vi "Modify G08.vi"(7 "DG Number":i32, 8 "error in (no error)":errorcluster, 11 "Settings 2":T1={"Channel A"={"Delay (µs)"=0.013000000000000001, "Pulse Width (µs)"=0.019, "Output Modulo"=300, "Output Offset"=0, "Go Signal"=16, "Polarity"=TRUE, "Terminate"=FALSE}, "Channel B"={"Delay (µs)"=0.032, "Pulse Width (µs)"=0.019, "Output Modulo"=300, "Output Offset"=0, "Go Signal"=16, "Polarity"=TRUE, "Terminate"=FALSE}, "Channel C"={"Delay (µs)"=0.0, "Pulse Width (µs)"=0.01, "Output Modulo"=300, "Output Offset"=0, "Go Signal"=16, "Polarity"=TRUE, "Terminate"=FALSE}, "Channel D"={"Delay (µs)"=0.01, "Pulse Width (µs)"=0.01, "Output Modulo"=300, "Output Offset"=0, "Go Signal"=16, "Polarity"=TRUE, "Terminate"=FALSE}, "Channel E"={"Delay (µs)"=0.039999999999999994, "Pulse Width (µs)"=0.01, "Output Modulo"=300, "Output Offset"=1, "Go Signal"=16, "Polarity"=TRUE, "Terminate"=FALSE, "Disconnect"=FALSE, "Onto MsBus"=FALSE, "Input Positive"=TRUE}, "Channel F"={"Delay (µs)"=0.04999999999999999, "Pulse Width (µs)"=0.01, "Output Modulo"=300, "Output Offset"=1, "Go Signal"=16, "Polarity"=TRUE, "Terminate"=FALSE, "Disconnect"=FALSE, "Onto MsBus"=FALSE, "Input Positive"=TRUE}, "Clock Enable"=TRUE, "Ocillator Divider"=2, "Trigger Divider"=1, "Trigger Multiplier"=4, "Clock Source"=3, "Trigger Terminate"=TRUE, "Gate Terminate"=TRUE, "Trigger Level"=0.2, "Gate Level"=0.0, "Gate Delay (µs)"=-1.0, "MS Bus"=1, "Internal Clock (µs)"=0.0083333, "Stop Trigger"=1, "Gate Divider"=0, "Force Trigger (µs)"=-1.0, "Step Back Time (µs)"=-1.0, "Burst Counter"=1, "Positive Gate"=TRUE, "Trigger Source"=TRUE, "Gate Type"=TRUE, "Synchronize Gate"=FALSE, "Trigger Slope"=TRUE, "Stop on Preset"=FALSE, "Reset When Done"=TRUE, "Trigger Enable"=TRUE, "Gate AB"=0, "Gate CD"=0, "Gate EF"=0} {"Gate EF" items=["Normal"=0, "EF_OR"=1048576, "EF_AND"=2097152, "EF_XOR"=3145728]; "Gate CD" items=["Normal"=0, "CD_OR"=262144, "CD_AND"=524288, "CD_XOR"=786432]; "Gate AB" items=["Normal"=0, "AB_OR"=65536, "AB_AND"=131072, "AB_XOR"=196608]; "Step Back Time (µs)" min=-1.0 format="%.6f"; "Force Trigger (µs)" min=-1.0 format="%.6f"; "Gate Delay (µs)" min=-1.0 format="%.6f"; "Internal Clock (µs)" min=0.0 format="%.6f"; "MS Bus" format="%04x" items=["Local Primary"=1, "Local Secondary"=2, "Local Force"=4, "Resynchronize"=8, "Master Primary"=16, "Master Secondary"=32, "Master Force"=64, "System Clock"=128, "Delay Clock"=256, "Inhibit Local"=512, "Start Local"=1024, "Start Bus"=2048, "Step Back Local"=4096, "Step Back Bus"=8192, "Enable From E"=65536, "Enable From F"=131072, "Enable From Bus"=262144]; "Gate Level" min=-2.5 max=2.5 format="%.3g"; "Trigger Level" min=-2.5 max=2.5 format="%.3f"; "Clock Source" items=["Internal Oscillator"=1, "External Trigger"=2, "Trigger & Oscillator"=3, "Master Slave Bus"=4]; "Trigger Multiplier" min=1; "Trigger Divider" min=1; "Ocillator Divider" min=1; "Channel F"."Go Signal" format="%04x" items=["Loc Prim"=1, "Loc Sec"=2, "Loc Force"=4, "Resynch"=8, "Mas Prim"=16, "Mas Sec"=32, "Mas Force"=64, "Sys Clock"=128, "Delay Clock"=256, "Inhibit Local"=512, "Start Local"=1024, "Start Bus"=2048, "Step Back Loc"=4096, "Step Back Bus"=8192, "From E"=65536, "From F"=131072, "From Bus"=262144]; "Channel F"."Pulse Width (µs)" min=0.0 max=8947840.0 format="%.6f"; "Channel F"."Delay (µs)" min=0.0 format="%.6f"; "Channel E"."Go Signal" format="%04x" items=["Loc Prim"=1, "Loc Sec"=2, "Loc Force"=4, "Resynch"=8, "Mas Prim"=16, "Mas Sec"=32, "Mas Force"=64, "Sys Clock"=128, "Delay Clock"=256, "Inhibit Local"=512, "Start Local"=1024, "Start Bus"=2048, "Step Back Loc"=4096, "Step Back Bus"=8192, "From E"=65536, "From F"=131072, "From Bus"=262144]; "Channel E"."Pulse Width (µs)" min=0.0 max=8947840.0 format="%.6f"; "Channel E"."Delay (µs)" min=0.0 format="%.6f"; "Channel D"."Go Signal" format="%04x" items=["Loc Prim"=1, "Loc Sec"=2, "Loc Force"=4, "Resynch"=8, "Mas Prim"=16, "Mas Sec"=32, "Mas Force"=64, "Sys Clock"=128, "Delay Clock"=256, "Inhibit Local"=512, "Start Local"=1024, "Start Bus"=2048, "Step Back Loc"=4096, "Step Back Bus"=8192, "From E"=65536, "From F"=131072, "From Bus"=262144]; "Channel D"."Pulse Width (µs)" min=0.0 max=8947840.0 format="%.6f"; "Channel D"."Delay (µs)" min=0.0 format="%.6f"; "Channel C"."Go Signal" format="%04x" items=["Loc Prim"=1, "Loc Sec"=2, "Loc Force"=4, "Resynch"=8, "Mas Prim"=16, "Mas Sec"=32, "Mas Force"=64, "Sys Clock"=128, "Delay Clock"=256, "Inhibit Local"=512, "Start Local"=1024, "Start Bus"=2048, "Step Back Loc"=4096, "Step Back Bus"=8192, "From E"=65536, "From F"=131072, "From Bus"=262144]; "Channel C"."Pulse Width (µs)" min=0.0 max=8947840.0 format="%.6f"; "Channel C"."Delay (µs)" min=0.0 format="%.6f"; "Channel B"."Go Signal" format="%04x" items=["Loc Prim"=1, "Loc Sec"=2, "Loc Force"=4, "Resynch"=8, "Mas Prim"=16, "Mas Sec"=32, "Mas Force"=64, "Sys Clock"=128, "Delay Clock"=256, "Inhibit Local"=512, "Start Local"=1024, "Start Bus"=2048, "Step Back Loc"=4096, "Step Back Bus"=8192, "From E"=65536, "From F"=131072, "From Bus"=262144]; "Channel B"."Pulse Width (µs)" min=0.0 max=8947840.0 format="%.6f"; "Channel B"."Delay (µs)" min=0.0 format="%.6f"; "Channel A"."Go Signal" format="%04x" items=["Loc Prim"=1, "Loc Sec"=2, "Loc Force"=4, "Resynch"=8, "Mas Prim"=16, "Mas Sec"=32, "Mas Force"=64, "Sys Clock"=128, "Delay Clock"=256, "Inhibit Local"=512, "Start Local"=1024, "Start Bus"=2048, "Step Back Loc"=4096, "Step Back Bus"=8192, "From E"=65536, "From F"=131072, "From Bus"=262144]; "Channel A"."Pulse Width (µs)" min=0.0 max=8947840.0 format="%.6f"; "Channel A"."Delay (µs)" min=0.0 format="%.6f"}) -> (0 "error out":errorcluster)   [LabVIEW 2009, in "POLARIS BME DG.lvlib"]
doc: "long Set_BME_G05(double FireFirst_T0, unsigned long OutputModulo_T0, BOOL Active_T0, BOOL Positive_T0, BOOL Terminate_T0, BOOL HighDrive_T0, double FireFirst_A, unsigned long OutputModulo_A, BOOL Active_A, BOOL Positive_A, BOOL Terminate_A, BOOL HighDrive_A, double FireFirst_B, unsigned long OutputModulo_B, BOOL Active_B, BOOL Positive_B, BOOL Terminate_B, BOOL HighDrive_B, BOOL Gate_AB, unsigned long OutputLevel, BOOL TriggerTerminate, BOOL ClockEnable, double InternalClock, double TriggerLevel, unsigned long PresetValue, unsigned long DivideBy, unsigned long ClockSource, unsigned long GateDivider, BOOL PositiveGate, BOOL InternalTrigger, BOOL InternalArm, BOOL SoftwareTrigger, BOOL RisingEdge, BOOL StopOnPreset, BOOL ResetWhenDone, BOOL TriggerEnable, long DG_Number);"
uses:
  POLARIS BME DG.lvlib
  Settings G08.ctl
  BME DLL/DelayGenerator.dll
panel:
  # "NOTICE -- YOU MUST LEAVE THIS NOTICE IN PLACE.  PER THE TERMS OF THE LICENSE BELOW, YOU MAY SUBLICENSE THIS SOFTWARE \nIN ANY WAY THAT DOES NOT CONFLICT WITH THIS LICENSE.\n\n### BSD License (http://www.opensource.org/licenses/bsd-license.php) Begin ###\n \nCopyright (c) 2011, Applied Energetics, http://www.appliedenergetics.com,\n                               Richard Schwerdtfeger, <rschwerdtfeger@appliedenergetics.com>\n\nAll rights reserved.\n\nRedistribution and use in source and binary forms, with or without modification, are permitted provided that the \nfollowing conditions are met:\n\n    * Redistributions of source code must retain the above copyright notice, this list of conditions and the following disclaimer.\n    * Redistributions in binary form must reproduce the above copyright notice, this list of conditions and the following disclaimer \n       in the documentation and/or other materials provided with the distribution.\n    * Neither the name of Richard Schwerdtfeger, Applied Energetics, Inc., nor the names of its contributors may be used to \n       endorse or promote products derived from this software without specific prior written permission.\n\nTHIS SOFTWARE IS PROVIDED BY THE COPYRIGHT HOLDERS AND CONTRIBUTORS \"AS IS\" AND ANY EXPRESS OR IMPLIED WARRANTIES, \nINCLUDING, BUT NOT LIMITED TO, THE IMPLIED WARRANTIES OF MERCHANTABILITY AND FITNESS FOR A PARTICULAR PURPOSE ARE \nDISCLAIMED. IN NO EVENT SHALL THE COPYRIGHT OWNER OR CONTRIBUTORS BE LIABLE FOR ANY DIRECT, INDIRECT, INCIDENTAL,\n SPECIAL, EXEMPLARY, OR CONSEQUENTIAL DAMAGES (INCLUDING, BUT NOT LIMITED TO, PROCUREMENT OF SUBSTITUTE GOODS OR \nSERVICES; LOSS OF USE, DATA, OR PROFITS; OR BUSINESS INTERRUPTION) HOWEVER CAUSED AND ON ANY THEORY OF LIABILITY, \nWHETHER IN CONTRACT, STRICT LIABILITY, OR TORT (INCLUDING NEGLIGENCE OR OTHERWISE) ARISING IN ANY WAY OUT OF THE USE \nOF THIS SOFTWARE, EVEN IF ADVISED OF THE POSSIBILITY OF SUCH DAMAGE.\n\n### BSD License End ###"
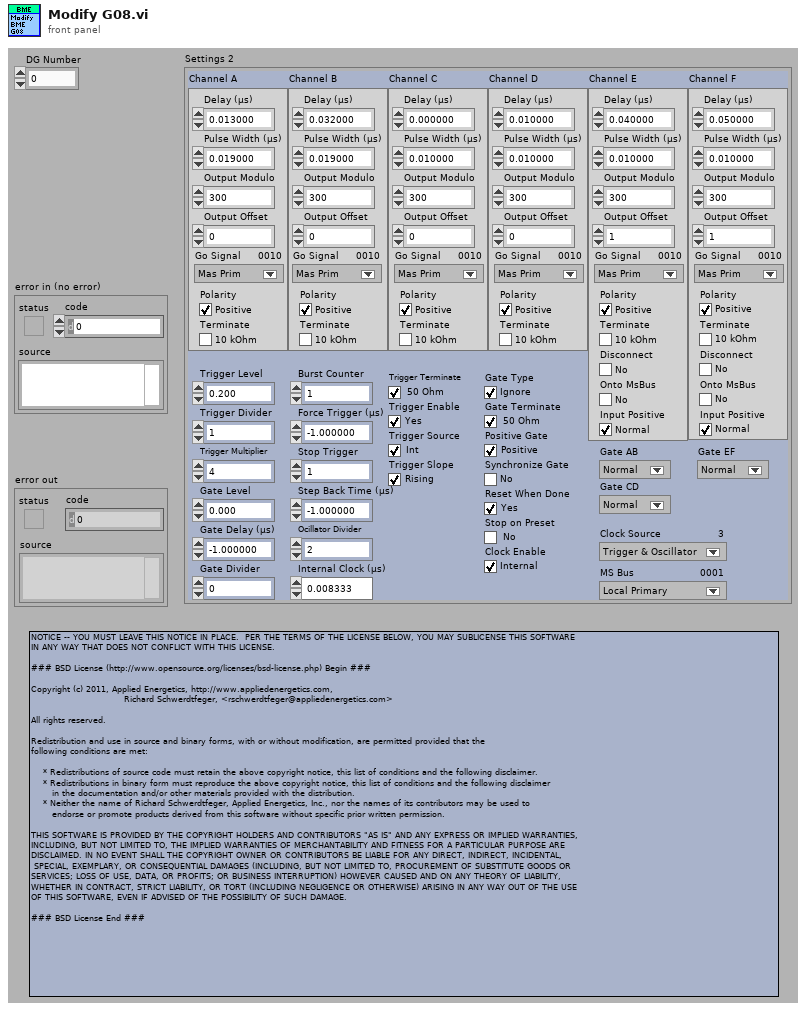
[diagram p1: front panel]
types:
  T1 = typedef "POLARIS BME DG.lvlib/Settings G08.ctl" = cluster{"Channel A":cluster{"Delay (µs)":dbl, "Pulse Width (µs)":dbl, "Output Modulo":u32, "Output Offset":u32, "Go Signal":u32, "Polarity":bool, "Terminate":bool}, "Channel B":cluster{"Delay (µs)":dbl, "Pulse Width (µs)":dbl, "Output Modulo":u32, "Output Offset":u32, "Go Signal":u32, "Polarity":bool, "Terminate":bool}, "Channel C":cluster{"Delay (µs)":dbl, "Pulse Width (µs)":dbl, "Output Modulo":u32, "Output Offset":u32, "Go Signal":u32, "Polarity":bool, "Terminate":bool}, "Channel D":cluster{"Delay (µs)":dbl, "Pulse Width (µs)":dbl, "Output Modulo":u32, "Output Offset":u32, "Go Signal":u32, "Polarity":bool, "Terminate":bool}, "Channel E":cluster{"Delay (µs)":dbl, "Pulse Width (µs)":dbl, "Output Modulo":u32, "Output Offset":u32, "Go Signal":u32, "Polarity":bool, "Terminate":bool, "Disconnect":bool, "Onto MsBus":bool, "Input Positive":bool}, "Channel F":cluster{"Delay (µs)":dbl, "Pulse Width (µs)":dbl, "Output Modulo":u32, "Output Offset":u32, "Go Signal":u32, "Polarity":bool, "Terminate":bool, "Disconnect":bool, "Onto MsBus":bool, "Input Positive":bool}, "Clock Enable":bool, "Ocillator Divider":u32, "Trigger Divider":u32, "Trigger Multiplier":u32, "Clock Source":u32, "Trigger Terminate":bool, "Gate Terminate":bool, "Trigger Level":dbl, "Gate Level":dbl, "Gate Delay (µs)":dbl, "MS Bus":u32, "Internal Clock (µs)":dbl, "Stop Trigger":u32, "Gate Divider":u32, "Force Trigger (µs)":dbl, "Step Back Time (µs)":dbl, "Burst Counter":u32, "Positive Gate":bool, "Trigger Source":bool, "Gate Type":bool, "Synchronize Gate":bool, "Trigger Slope":bool, "Stop on Preset":bool, "Reset When Done":bool, "Trigger Enable":bool, "Gate AB":u32, "Gate CD":u32, "Gate EF":u32}
  T2 = cluster{"Delay (µs)":dbl, "Pulse Width (µs)":dbl, "Output Modulo":u32, "Output Offset":u32, "Go Signal":u32, "Polarity":bool, "Terminate":bool}
  T3 = cluster{"Delay (µs)":dbl, "Pulse Width (µs)":dbl, "Output Modulo":u32, "Output Offset":u32, "Go Signal":u32, "Polarity":bool, "Terminate":bool, "Disconnect":bool, "Onto MsBus":bool, "Input Positive":bool}
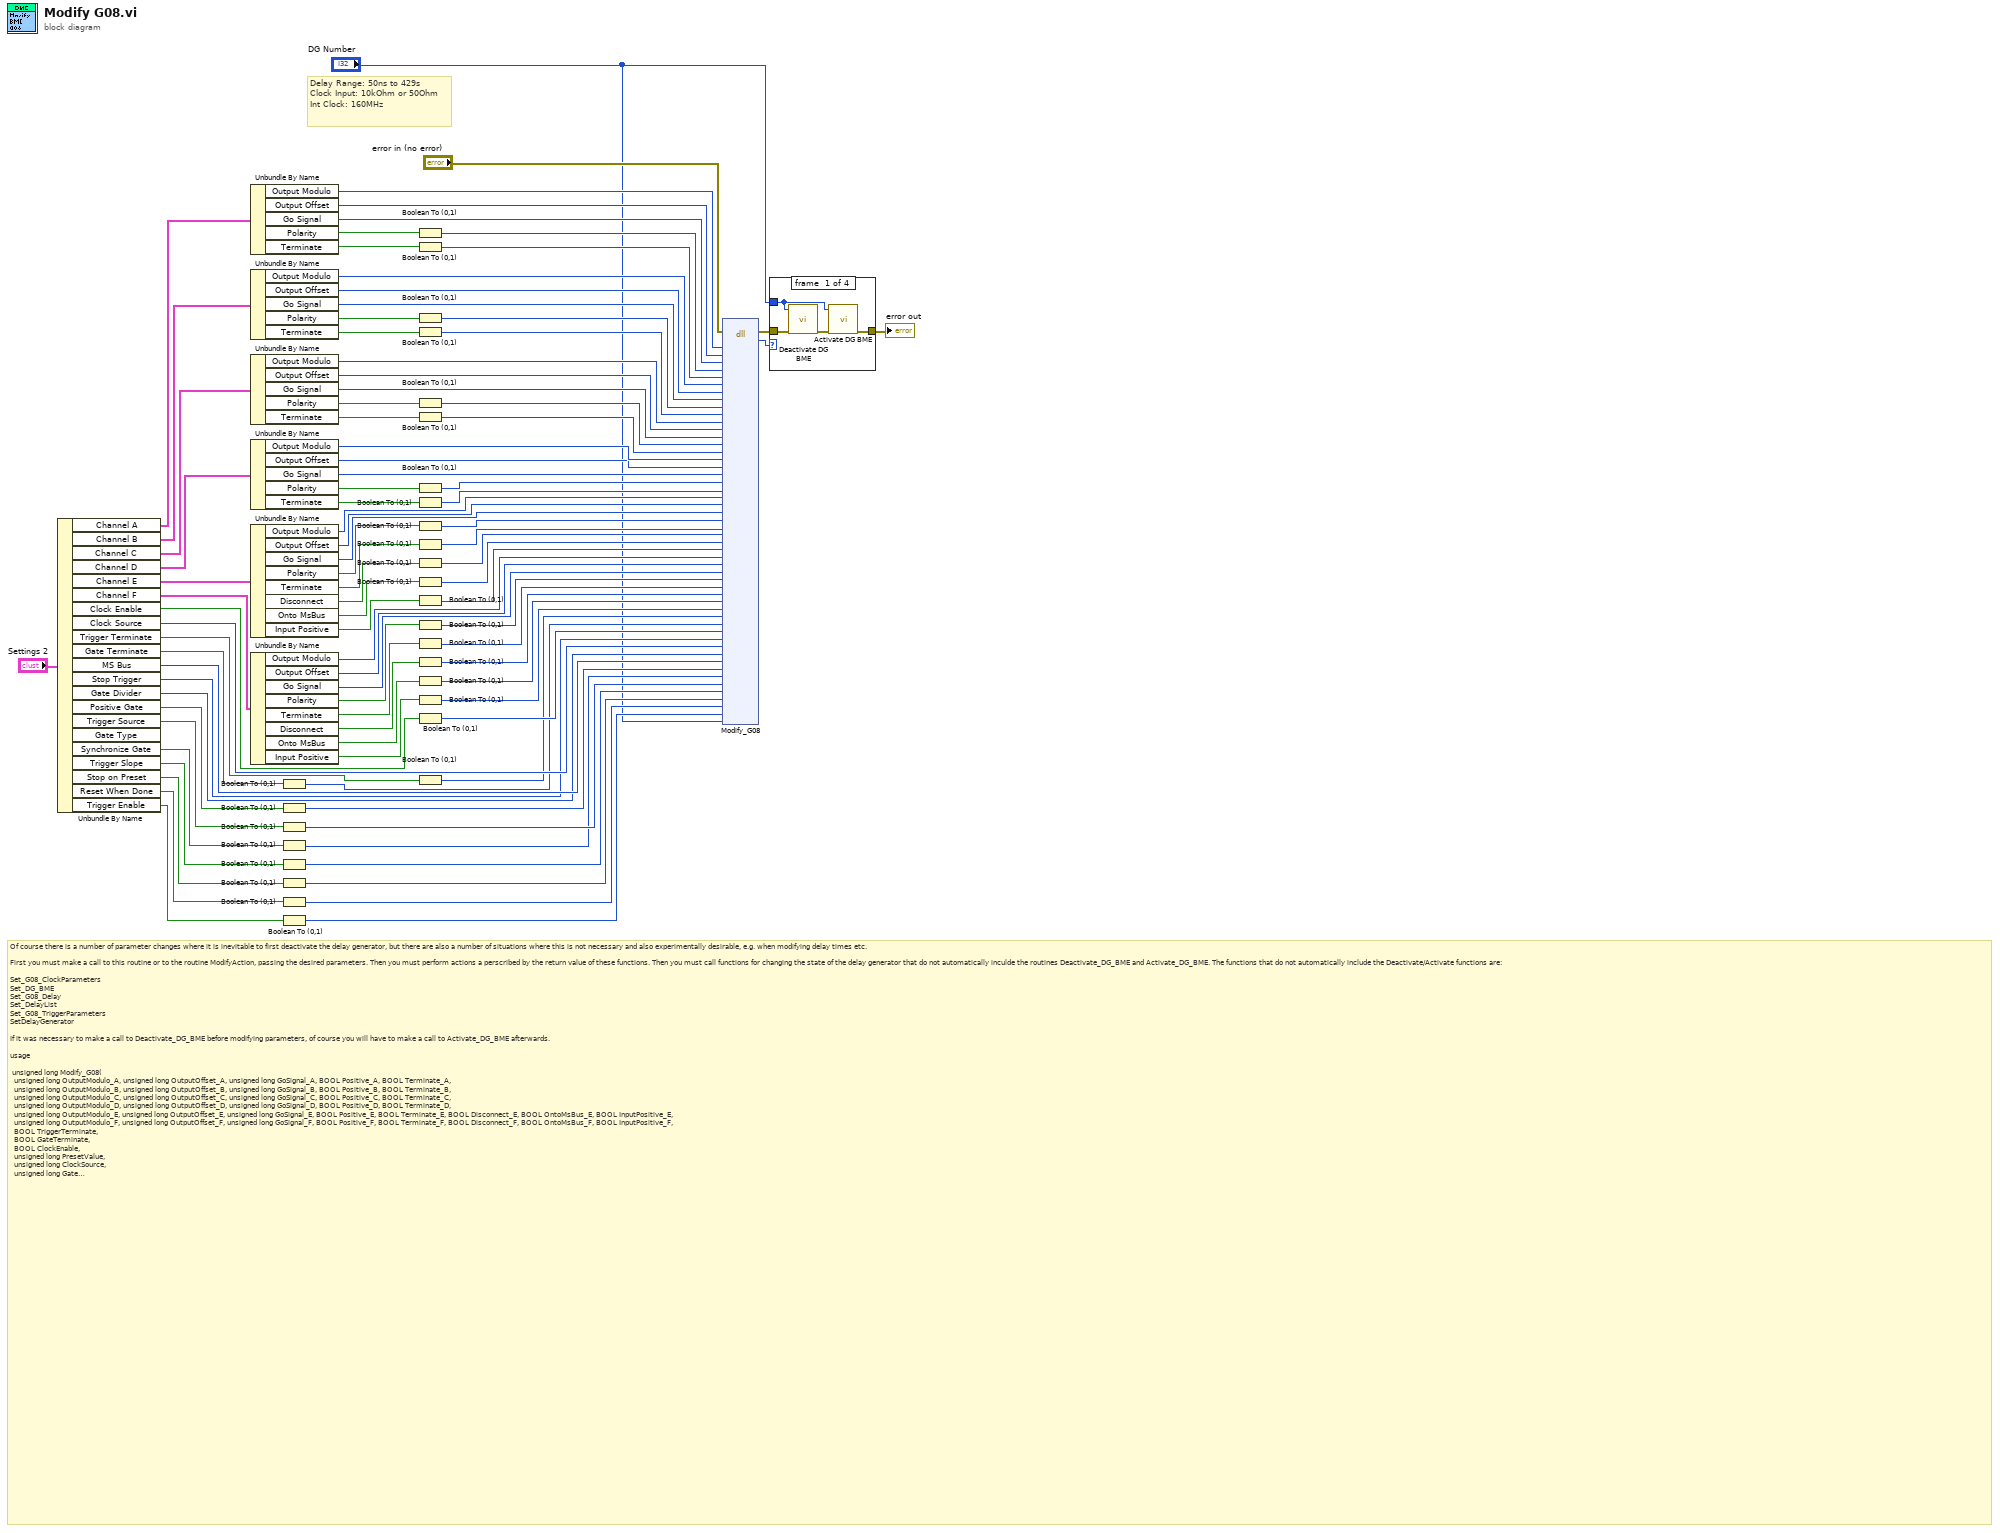
[diagram p0: block diagram]
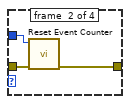
[diagram p2: hidden frame]
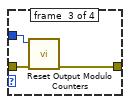
[diagram p3: hidden frame]
diagram:
  # "Delay Range: 50ns to 429s\nClock Input: 10kOhm or 50Ohm\nInt Clock: 160MHz"
  # "Of course there is a number of parameter changes where it is inevitable to first deactivate the delay generator, but there are also a number of situations where this is not necessary and also experimentally desirable, e.g. when modifying delay times etc. \n\nFirst you must make a call to this routine or to the routine ModifyAction, passing the desired parameters. Then you must perform actions a perscribed by the return value of these functions. Then you must call functions for changing the state of the delay generator that do not automatically inculde the routines Deactivate_DG_BME and Activate_DG_BME. The functions that do not automatically include the Deactivate/Activate functions are:\n\nSet_G08_ClockParameters\nSet_DG_BME\nSet_G08_Delay\nSet_DelayList\nSet_G08_TriggerParameters\nSetDelayGenerator\n\nIf it was necessary to make a call to Deactivate_DG_BME before modifying parameters, of course you will have to make a call to Activate_DG_BME afterwards.\n\nusage\n\n\tunsigned long Modify_G08(\n\t\tunsigned long OutputModulo_A, unsigned long OutputOffset_A, unsigned long GoSignal_A, BOOL Positive_A, BOOL Terminate_A,\n\t\tunsigned long OutputModulo_B, unsigned long OutputOffset_B, unsigned long GoSignal_B, BOOL Positive_B, BOOL Terminate_B,\n\t\tunsigned long OutputModulo_C, unsigned long OutputOffset_C, unsigned long GoSignal_C, BOOL Positive_C, BOOL Terminate_C,\n\t\tunsigned long OutputModulo_D, unsigned long OutputOffset_D, unsigned long GoSignal_D, BOOL Positive_D, BOOL Terminate_D,\n\t\tunsigned long OutputModulo_E, unsigned long OutputOffset_E, unsigned long GoSignal_E, BOOL Positive_E, BOOL Terminate_E, BOOL Disconnect_E, BOOL OntoMsBus_E, BOOL InputPositive_E, \n\t\tunsigned long OutputModulo_F, unsigned long OutputOffset_F, unsigned long GoSignal_F, BOOL Positive_F, BOOL Terminate_F, BOOL Disconnect_F, BOOL OntoMsBus_F, BOOL InputPositive_F, \n\t\tBOOL TriggerTerminate, \n\t\tBOOL GateTerminate, \n\t\tBOOL ClockEnable,\n\t\tunsigned long PresetValue,\n\t\tunsigned long ClockSource, \n\t\tunsigned long GateDivider,\n\t\tunsigned long MS_Bus, \n\t\tBOOL PositiveGate, \n\t\tBOOL SynchronizeGate,\n\t\tBOOL InternalTrigger, \n\t\tBOOL RisingEdge, \n\t\tBOOL StopOnPreset,\n\t\tBOOL ResetWhenDone, \n\t\tBOOL TriggerEnable, \n\t\tlong DG_Number);\n\nparameters\n\n\tSee the above named routines, e.g. Set_G08_TriggerParameters for a description of the parameters. Note that this routine does not pass the complete set of parameters, since for some parameters there is no action necessary under any situation.\n\nreturn value\n\n\tThe return value of this function indicates the actions that are also necessary when the specified parameters are to be set. Each bit in the return value specifies an action that should be performed:\n\tBit 0 True:  it is necessary to call the routine Deactivate_DG_BME before actually calling the routine SetDelayGenerator.\n\tBit 1 True:  it is necessary to call the routine ResetEventCounter.\n\tBit 2 True:  it is necessary to call the routine ResetOutputModuloCounters."
  n1 = Unbundle By Name("Settings 2") -> ("Channel A"=w80:T2, "Channel B"=w67:T2, "Channel C"=w66:T2, "Channel D"=w65:T2, "Channel E"=w64:T3, "Channel F"=w63:T3, "Clock Enable"=w81:bool, "Clock Source"=w31:u32, "Trigger Terminate"=w82:bool, "Gate Terminate"=w83:bool, "MS Bus"=w28:u32, "Stop Trigger"=w27:u32, "Gate Divider"=w26:u32, "Positive Gate"=w84:bool, "Trigger Source"=w85:bool, "Synchronize Gate"=w86:bool, "Trigger Slope"=w87:bool, "Stop on Preset"=w88:bool, "Reset When Done"=w89:bool, "Trigger Enable"=w90:bool)  [unwired: 1 out]
  n2 = Unbundle By Name(w80) -> ("Output Modulo"=w62:u32, "Output Offset"=w61:u32, "Go Signal"=w60:u32, "Polarity"=w79:bool, "Terminate"=w78:bool)
  n3 = Unbundle By Name(w67) -> ("Output Modulo"=w57:u32, "Output Offset"=w56:u32, "Go Signal"=w55:u32, "Polarity"=w76:bool, "Terminate"=w77:bool)
  n4 = Unbundle By Name(w66) -> ("Output Modulo"=w52:u32, "Output Offset"=w51:u32, "Go Signal"=w50:u32, "Polarity"=w72:bool, "Terminate"=w73:bool)
  n5 = Unbundle By Name(w65) -> ("Output Modulo"=w47:u32, "Output Offset"=w46:u32, "Go Signal"=w45:u32, "Polarity"=w75:bool, "Terminate"=w74:bool)
  n6 = Unbundle By Name(w64) -> ("Output Modulo"=w42:u32, "Output Offset"=w41:u32, "Go Signal"=w40:u32, "Polarity"=w71:bool, "Terminate"=w70:bool, "Disconnect"=w18:bool, "Onto MsBus"=w17:bool, "Input Positive"=w16:bool)
  n7 = Unbundle By Name(w63) -> ("Output Modulo"=w37:u32, "Output Offset"=w36:u32, "Go Signal"=w35:u32, "Polarity"=w68:bool, "Terminate"=w69:bool, "Disconnect"=w12:bool, "Onto MsBus"=w11:bool, "Input Positive"=w10:bool)
  n8 = Boolean To (0,1)(Boolean=w83) -> (0, 1=w29:i16)
  n9 = Boolean To (0,1)(Boolean=w84) -> (0, 1=w25:i16)
  n10 = Boolean To (0,1)(Boolean=w85) -> (0, 1=w24:i16)
  n11 = Boolean To (0,1)(Boolean=w86) -> (0, 1=w23:i16)
  n12 = Boolean To (0,1)(Boolean=w87) -> (0, 1=w22:i16)
  n13 = Boolean To (0,1)(Boolean=w88) -> (0, 1=w21:i16)
  n14 = Boolean To (0,1)(Boolean=w89) -> (0, 1=w20:i16)
  n15 = Boolean To (0,1)(Boolean=w90) -> (0, 1=w19:i16)
  n16 = Boolean To (0,1)(Boolean=w79) -> (0, 1=w59:i16)
  n17 = Boolean To (0,1)(Boolean=w78) -> (0, 1=w58:i16)
  n18 = Boolean To (0,1)(Boolean=w76) -> (0, 1=w54:i16)
  n19 = Boolean To (0,1)(Boolean=w77) -> (0, 1=w53:i16)
  n20 = Boolean To (0,1)(Boolean=w72) -> (0, 1=w49:i16)
  n21 = Boolean To (0,1)(Boolean=w73) -> (0, 1=w48:i16)
  n22 = Boolean To (0,1)(Boolean=w75) -> (0, 1=w44:i16)
  n23 = Boolean To (0,1)(Boolean=w74) -> (0, 1=w43:i16)
  n24 = Boolean To (0,1)(Boolean=w71) -> (0, 1=w39:i16)
  n25 = Boolean To (0,1)(Boolean=w70) -> (0, 1=w38:i16)
  n26 = Boolean To (0,1)(Boolean=w18) -> (0, 1=w13:i16)
  n27 = Boolean To (0,1)(Boolean=w17) -> (0, 1=w14:i16)
  n28 = Boolean To (0,1)(Boolean=w16) -> (0, 1=w15:i16)
  n29 = Boolean To (0,1)(Boolean=w68) -> (0, 1=w34:i16)
  n30 = Boolean To (0,1)(Boolean=w69) -> (0, 1=w33:i16)
  n31 = Boolean To (0,1)(Boolean=w12) -> (0, 1=w7:i16)
  n32 = Boolean To (0,1)(Boolean=w11) -> (0, 1=w8:i16)
  n33 = Boolean To (0,1)(Boolean=w10) -> (0, 1=w9:i16)
  n34 = Boolean To (0,1)(Boolean=w81) -> (0, 1=w32:i16)
  n35 = Boolean To (0,1)(Boolean=w82) -> (0, 1=w30:i16)
  n36 = dll-call lib="C:/CS Framework/LVSCC/LV2009/GPL/Projects/cs-framework/CSClass/CSPOLARIS/POLARIS BME DG/BME DLL/DelayGenerator.dll" fn="Modify_G08"(error in="error in (no error)", "OutputModulo_A"=w62, "OutputOffset_A"=w61, "GoSignal_A"=w60, "Positive_A"=w59, "Terminate_A"=w58, "OutputModulo_B"=w57, "OutputOffset_B"=w56, "GoSignal_B"=w55, "Positive_B"=w54, "Terminate_B"=w53, "OutputModulo_C"=w52, "OutputOffset_C"=w51, "GoSignal_C"=w50, "Positive_C"=w49, "Terminate_C"=w48, "OutputModulo_D"=w47, "OutputOffset_D"=w46, "GoSignal_D"=w45, "Positive_D"=w44, "Terminate_D"=w43, "OutputModulo_E"=w42, "OutputOffset_E"=w41, "GoSignal_E"=w40, "Positive_E"=w39, "Terminate_E"=w38, "Disconnect_E"=w13, "OntoMsBus_E"=w14, "InputPositive_E"=w15, "OutputModulo_F"=w37, "OutputOffset_F"=w36, "GoSignal_F"=w35, "Positive_F"=w34, "Terminate_F"=w33, "Disconnect_F"=w7, "OntoMsBus_F"=w8, "InputPositive_F"=w9, "TriggerTerminate"=w30, "GateTerminate"=w29, "ClockEnable"=w32, "PresetValue"=w27, "ClockSource"=w31, "GateDivider"=w26, "MS_Bus"=w28, "PositiveGate"=w25, "SynchronizeGate"=w23, "InternalTrigger"=w24, "RisingEdge"=w22, "StopOnPreset"=w21, "ResetWhenDone"=w20, "TriggerEnable"=w19, "DG_Number"="DG Number") -> (error out=w3:errorcluster, "return type"=w4:i32)  [unwired: 53 in, 1 out]
  n37 = case shown="1" w4 {
    tunnel: w3 -> [w94 w97 w100 w101]
    tunnel: [w92 w96 w99 w101] -> w2
    tunnel: "DG Number" -> [w91 w95 w98 _]
    frame #0 {
      n38 = call "Deactivate DG BME.vi"("error in (no error)"=w94, "DG Number"=w91) -> ("error out"=w93:errorcluster)  [unwired: 9 out]
      n39 = call "Activate DG BME.vi"("error in (no error)"=w93, "DG Number"=w91) -> ("error out"=w92:errorcluster)  [unwired: 9 out]
    }
    frame #1 {
      n40 = call "Reset Event Counter.vi"("error in (no error)"=w97, "DG Number"=w95) -> ("error out"=w96:errorcluster)  [unwired: 9 out]
    }
    frame #2 {
      n41 = call "Reset Output Modulo Counters.vi"("error in (no error)"=w100, "DG Number"=w98) -> ("error out"=w99:errorcluster)  [unwired: 9 out]
    }
    frame #3 {
    }
  }
  "error out" <- w2
